vi "Choreo_ChoreoSwerve_LoadAllTrajectories.vi"(8 "error in (no error)":errorcluster) -> (0 "error out":errorcluster)   [LabVIEW 2019, in "ChoreoLib.lvlib"]
doc: "Load a Choreo trajectory from a JSON formatted file. Note that for newer versions of Choreo, the file has a \".traj\" extension. Internally this is formatted as a JSON file.\n\nInputs: \n - filename - string - The name of the trajectory file. See notes below on file naming.\n\nOutputs:\n - Trajectory - cluster - Trajectory read from JSON file.\n - Error out - cluster - Error cluster\n - Full Filename - string - fully qualified file name.\n\nNotes on file naming:\n - The file name must include the extention. \".json\", or \".traj\" is not automatically appended to the name. \n - The file name can be a simple file or an absolute path. If a simple file name is used the default path on the RoboRIO is: \"home:\\lvuser\\natinst\\LabVIEW Data\". On a Windows PC the default path is the LabVIEW default directory. Normally this is: “%HOMEDRIVE%%HOMEPATH%\\Documents\\LabView Data\".\n - Filenames on the RoboRIO, which runs Linux, are case sensitive."
uses:
  ChoreoLib.lvlib
panel:
  out "Trajectories":string[](array[string])
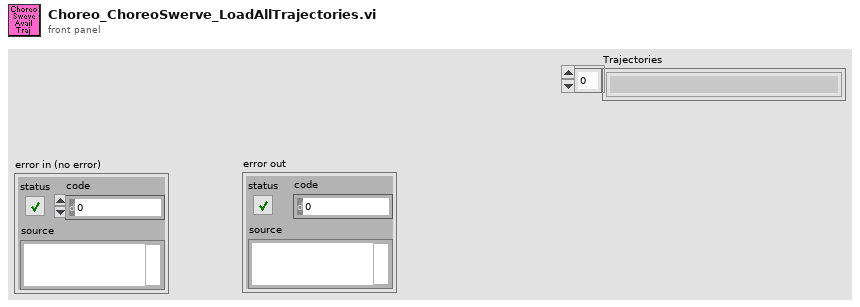
[diagram p1: front panel]
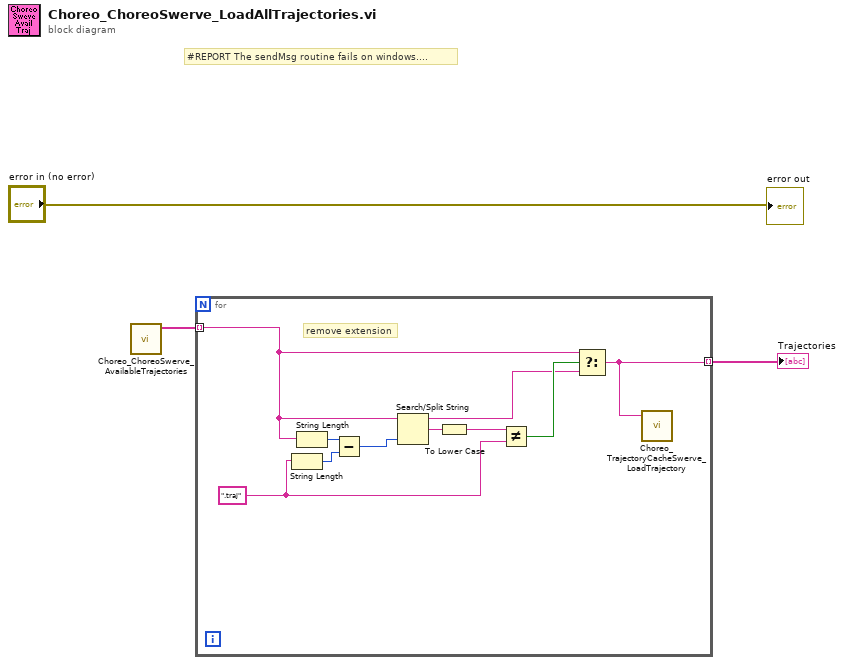
[diagram p0: block diagram]
diagram:
  # "#REPORT The sendMsg routine fails on windows...."
  n1 = call "Choreo_ChoreoSwerve_AvailableTrajectories.vi"() -> ("filenames"=w3:string[])  [unwired: 10 in, 1 out]
  n2 = for {
    tunnel: w3 -> [w6] mode=indexing
    tunnel: [w4] -> w2 mode=indexing
    w7 = ".traj" ("y")
    # "remove extension"
    n3 = String Length(string=w7) -> (length=w8:i32)
    n4 = String Length(string=w6) -> (length=w13:i32)
    n5 = Subtract(x=w13, y=w8) -> (x-y=w12:i32)
    n6 = Search/Split String(string=w6, offset (0)=w12) -> (substring before match=w5:string, match + rest of string=w11:string)  [unwired: 1 in, 1 out]
    n7 = To Lower Case(string=w11) -> (all lower case string=w10:string)
    n8 = Not Equal?(x=w10, y=w7) -> (x != y?=w9:bool)
    n9 = Select(t=w6, s=w9, f=w5) -> (s? t:f=w4:string)
    n10 = call "Choreo_TrajectoryCacheSwerve_LoadTrajectory.vi"("TrajectoryName"=w4) -> ()  [unwired: 9 in, 2 out]
  }
  "Trajectories" <- w2
  "error out" <- "error in (no error)"
